vi "error_messages_switch.vi"(0 "Error message type number":dbl) -> ()   [LabVIEW 2010]
uses:
  misc/error_messages_global.vi
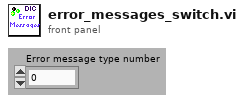
[diagram p1: front panel]
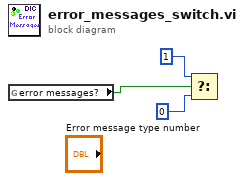
[diagram p0: block diagram]
diagram:
  n1 = global read "error_messages_global.vi" "error messages?"() -> (w1:bool)
  n2 = Select(t=1, s=w1, f=0) -> ()  [unwired: 1 out]
